vi "Chirp.vi"(4 "Beta/tao":fxp<+,52,48>=7000000000000.0, 6 "Beta":fxp<+,26,24>=7000000.0 format="%#.3p", 7 "first?":bool, 9 "Pulse width":u16, 10 "sign":bool, 11 "count":u16) -> (1 "Q":i16, 2 "I":i16, 3 "output valid":bool)   [LabVIEW 2017]
uses:
  <vilib>/rvi/FXPMathLib/FxpSinAndCos/subVIs/nifxpmath_SinAndCos_SimConfig.ctl
  <vilib>/rvi/FXPMathLib/FxpSinAndCos/simVIs/DllFxpSinAndCosTemp_sub.vi
  <vilib>/rvi/FXPMathLib/FxpMul/XNode/nifxpmath_Multiplier.xnode
  <vilib>/rvi/FXPMathLib/FxpSinAndCos/XNode/nifxpmath_SinAndCos.xnode
  <vilib>/rvi/FXPMathLib/sim/FxpSim.dll
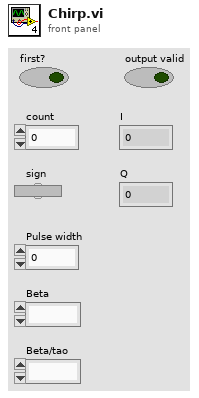
[diagram p1: front panel]
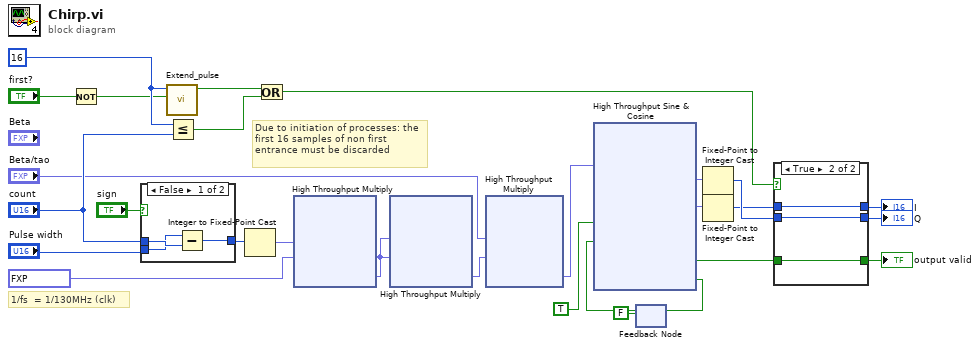
[diagram p0: block diagram]
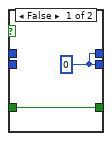
[diagram p2: hidden frame]
diagram:
  w23 = u16 16 ("x")
  # "1/fs  = 1/130MHz (clk)"
  # "Due to initiation of processes: the first 16 samples of non first entrance must be discarded"
  n1 = Not(x="first?") -> (.not. x?=w21:bool)
  n2 = case shown="False" "sign" {
    tunnel: [w29 w32] -> w20
    tunnel: "count" -> [w31 w32]
    tunnel: "Pulse width" -> [w30 _]
    frame False {
      n3 = Subtract(x=w30, y=w31) -> (x-y=w29:u16)
    }
    frame True {
    }
  }
  n4 = call "Extend_pulse.vi"("reset"=w21, "limit"=w23) -> ("pulse"=w22:bool)  [unwired: 9 in]
  n5 = Less Or Equal?(x=w23, y="count") -> (x <= y?=w8:bool)
  n6 = Integer to Fixed-Point Cast(integer=w20) -> (fixed-point=w16:fxp<+,16,16>)  [unwired: 1 in]
  n7 = Or(x=w22, y=w8) -> (x .or. y?=w1:bool)
  n8 = xnode ("High Throughput Multiply")("x"=w16, "y"=fxp<+,12,-18> 7.450580596923828e-09 ("1/fs")) -> ("x*y"=w17:fxp<+,28,-2>)
  n9 = xnode ("High Throughput Multiply")("x"=w17, "y"=w17) -> ("x*y"=w18:fxp<+,56,-4>)
  n10 = xnode ("High Throughput Multiply")("x"="Beta/tao", "y"=w18) -> ("x*y"=w19:fxp<+,32,4>)
  n11 = feedback #1(FALSE ("ready for input")) -> (w13:bool)
  n12 = xnode "High Throughput Sine & Cosine"("x (pi)"=w19, "input valid"=TRUE ("ready for output (T)"), "ready for output (T)"=w13) -> ("sin(x)"=w9:fxp<+/-,16,2>, "cos(x)"=w10:fxp<+/-,16,2>, "output valid"=w5:bool, "ready for input"=w12:bool)
  n13 = feedback-in #1(w12) -> ()
  n14 = Fixed-Point to Integer Cast(1:w9) -> (0:w7:i16)
  n15 = Fixed-Point to Integer Cast(1:w10) -> (0:w6:i16)
  n16 = case shown="True" w1 {
    tunnel: w7 -> [_ w35]
    tunnel: w6 -> [_ w37]
    tunnel: [w34 w37] -> w3
    tunnel: w5 -> [w33 w36]
    tunnel: [w33 w36] -> w4
    tunnel: [w34 w35] -> w2
    frame False {
      w34 = i16 0
    }
    frame True {
    }
  }
  "Q" <- w2
  "I" <- w3
  "output valid" <- w4
